vi "DELETEMEHandle setConfiguration.vi"(8 "error in (no error)":errorcluster, 10 "setConfiguration":variant, 11 "Inst.Krohn-Hite-7008 in":refnum<class "Inst.Krohn-Hite-7008.lvclass">) -> (0 "error out":errorcluster, 3 "Inst.Krohn-Hite-7008 out":refnum<class "Inst.Krohn-Hite-7008.lvclass">)   [LabVIEW 2019]
uses:
  45e4b271-6884-462c-ad3a-d505ab08eb62.vi
  Inst.Krohn-Hite-7008.lvclass
  C:/Program Files (x86)/National Instruments/LabVIEW 2019/user.lib/LevyLab/Instrument Framework/Instrument Types/VSource/Instrument.VSource.lvclass
  C:/Program Files (x86)/National Instruments/LabVIEW 2019/user.lib/LevyLab/Instrument Framework/SMOs/Instrument/Instrument.lvclass
  C:/Program Files (x86)/National Instruments/LabVIEW 2019/vi.lib/JKI/JKI SMO/SMO/SMO.lvclass
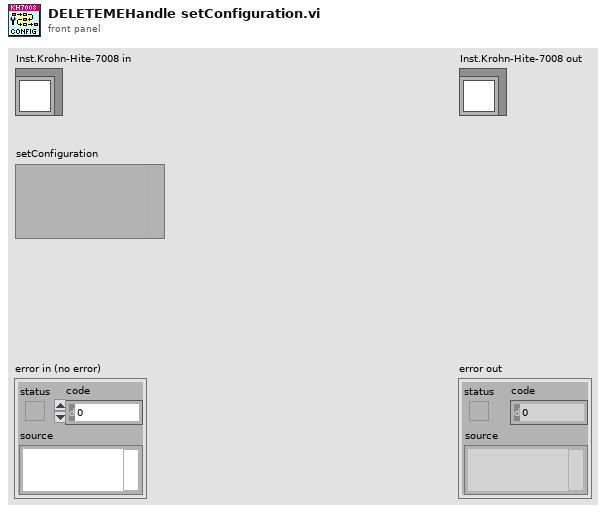
[diagram p1: front panel]
types:
  T1 = typedef "Inst.Krohn-Hite-7008.lvclass/Inst.Krohn-Hite-7008.Device--Cluster.ctl" = cluster{"Model":string, "device_id":string}
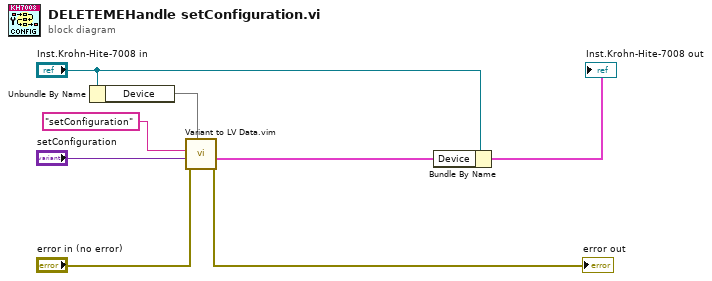
[diagram p0: block diagram]
diagram:
  n1 = Unbundle By Name("Inst.Krohn-Hite-7008 in") -> ("Device"=w7)
  n2 = call "Variant to LV Data.vim"("type"=w7, "error in (no error)"="error in (no error)", "JSON Data in"="setConfiguration", "Command"="setConfiguration") -> ("error out"=→"error out":errorcluster, "Data out"=w1:T1)  [unwired: 4 in, 2 out]
  n3 = Bundle By Name(cluster="Inst.Krohn-Hite-7008 in", "Device"=w1) -> (→"Inst.Krohn-Hite-7008 out":cluster{})
